vi "load template description map.vi"(11 "Path":path=path "D:/github/JKI-State-Machine-Plus/.doc/VI Description.md") -> (0 "Text":string, 2 "Array":string[](array[string]), 3 "Variant":variant)   [LabVIEW 2017]
uses:
  _tool/_file/csm-file-support.lvlib
  Communicable State Machine.lvlib
  _Shared/CSM Shared.lvlib
panel:
  out "values":string
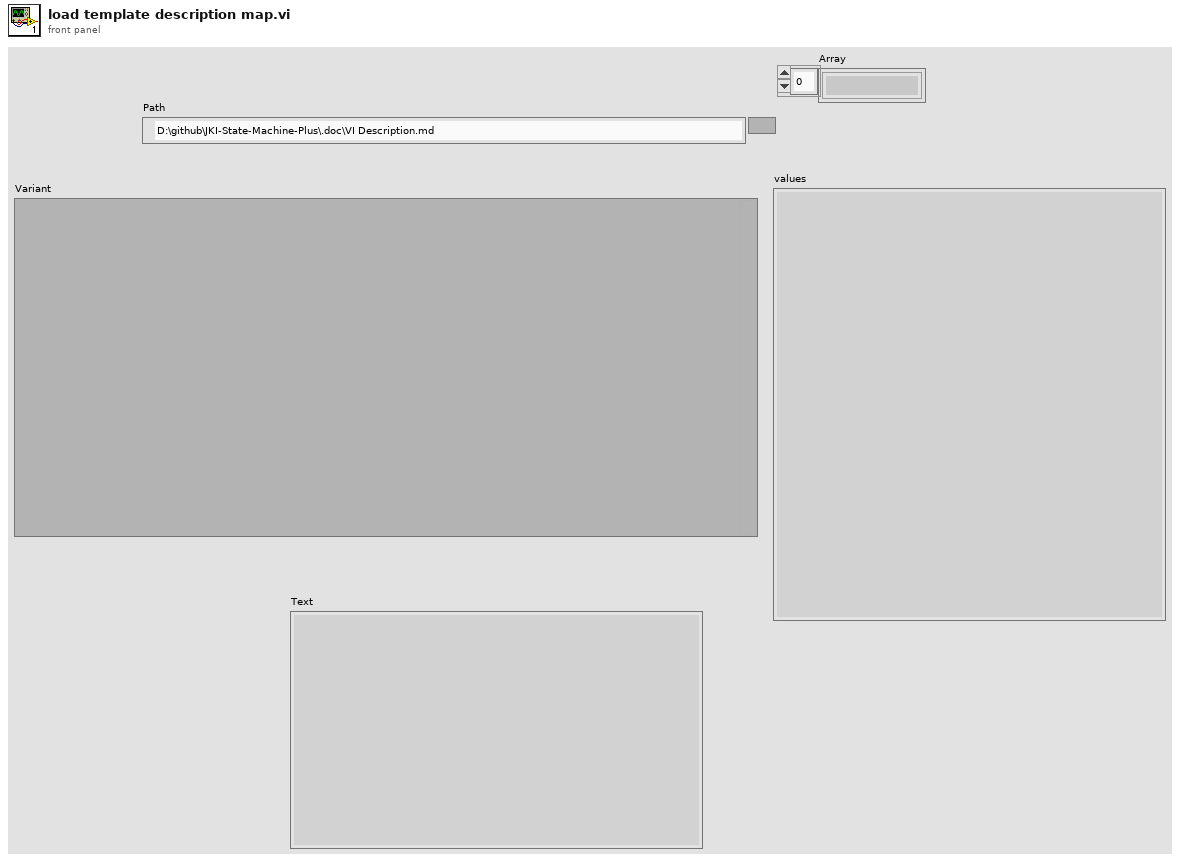
[diagram p1: front panel]
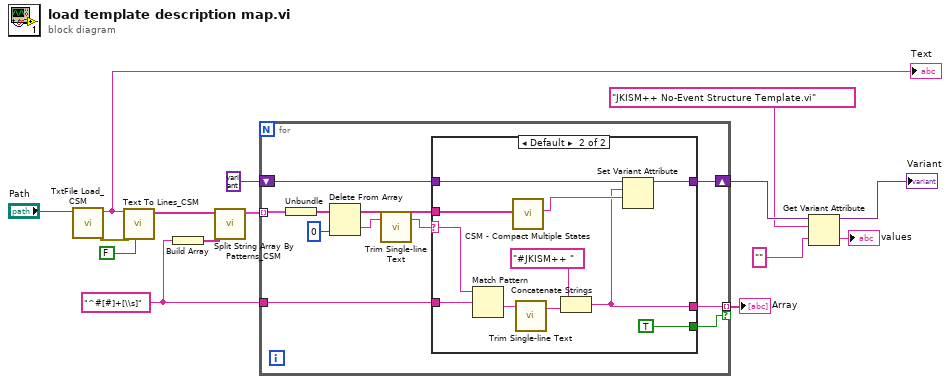
[diagram p0: block diagram]
diagram:
  w10 = "^#[#]+[\\s]" ("delimited string")
  n1 = call "TxtFile Load_CSM.vi"("Path"="Path") -> ("error out"=w14:errorcluster, "Text"=w13:string)  [unwired: 9 in]
  "Text" <- w13
  n2 = call "Text To Lines_CSM.vi"("Remove Empty Lines? (T)"=FALSE ("Remove Empty Lines?(T)"), "error in (no error)"=w14, "String"=w13) -> ("Lines"=w12:string[])  [unwired: 7 in, 1 out]
  n3 = Build Array(w10) -> (w9:string[])
  n4 = call "Split String Array By Patterns_CSM.vi"("Patterns"=w9, "Text Array"=w12) -> ("Array"=w11:cluster{"filtered array":string[]}[])  [unwired: 9 in]
  n5 = for {
    tunnel: w11 -> [w26] mode=indexing
    tunnel: w10 -> [w23]
    shift-right: [w20] -> w6
    shift-left: variant ("variant") -> [w21]
    tunnel: [w19] -> w1 mode=indexing if=w16
    n6 = Unbundle(w26) -> ("filtered array"=w25:string[])
    n7 = Delete From Array(array=w25, index=0) -> (deleted portion=w18:string, array with subset deleted=w22:string[])  [unwired: 1 in]
    n8 = call "Trim Single-line Text.vi"("single-line text"=w18) -> ("trimed text"=w17:string)  [unwired: 2 in]
    n9 = case shown="Default" w17 {
      selector: w17 -> [_ w29]
      tunnel: w23 -> [_ w38]
      tunnel: w22 -> [_ w36]
      tunnel: w21 -> [w27 w34]
      tunnel: [w27 w33] -> w20
      tunnel: [_ w31] -> w19
      tunnel: [_ TRUE] -> w16
      frame "" {
      }
      frame Default {
        n10 = Match Pattern(string=w29, regular expression=w38) -> (after substring=w37:string)  [unwired: 1 in, 3 out]
        n11 = call "CSM - Compact Multiple States.vi"("Multiple States"=w36) -> ("States"=w35:string)  [unwired: 9 in]
        n12 = call "Trim Single-line Text.vi"("single-line text"=w37) -> ("trimed text"=w32:string)  [unwired: 2 in]
        n13 = Concatenate Strings("#JKISM++ " ("string"), w32) -> (w31:string)
        n14 = Set Variant Attribute(Variant=w34, name=w31, value=w35) -> (Variant out=w33:variant)  [unwired: 1 in, 2 out]
      }
    }
  }
  "Array" <- w1
  n15 = Get Variant Attribute(Variant=w6, name="JKISM++ No-Event Structure Template.vi", default value (empty Variant)="" ("delimited string")) -> (duplicate Variant=→"Variant":variant, value=→"values":string)  [unwired: 1 in, 2 out]
